vi "TWM Client Cmd Exec ADC Selfcalibration.vi"(7 "end of packet key":string="TWM:command:EndOfPacket", 8 "error in":errorcluster, 10 "timeout [s] (300)":dbl=300.0, 11 "handle":i32) -> (0 "error out":errorcluster, 3 "handle out":i32)   [LabVIEW 2020, in "TWM Client.lvlib"]
doc: "Executes digitizer selfcalibration routine, waits for completion. It is blocking operation, so the client and TWM will hangup untill operation is done or fails! Cannot be called while measurement is in progress!"
uses:
  TWM Client.lvlib
  infolib.lvlib
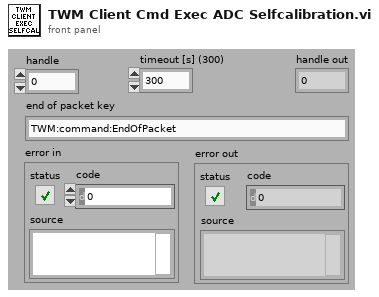
[diagram p1: front panel]
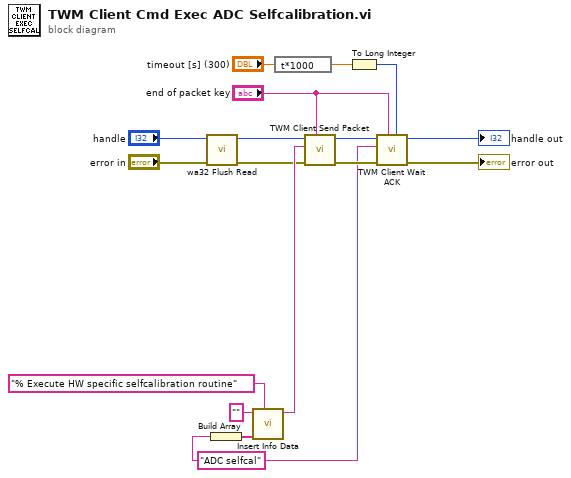
[diagram p0: block diagram]
diagram:
  w8 = "ADC selfcal" ("section name")
  n1 = call "wa32 Flush Read.vi"("error in"="error in", "handle"="handle") -> ("error out"=w3:errorcluster, "handle out"=w2:i32)  [unwired: 7 in, 1 out]
  n2 = Build Array(w8) -> (w16:string[])
  n3 = call "Insert Info Data.vi"("info data to insert"="% Execute HW specific selfcalibration routine", "sections"=w16, "info data"="") -> ("info data out"=w17:string)  [unwired: 7 in, 1 out]
  n4 = expression code="t*1000"("timeout [s] (300)") -> (w6:dbl)
  n5 = call "TWM Client Send Packet.vi"("end of packet key"="end of packet key", "error in"=w3, "command string"=w17, "handle"=w2) -> ("error out"=w14:errorcluster, "handle out"=w13:i32)  [unwired: 6 in]
  n6 = To Long Integer(number=w6) -> (32bit integer=w5:i32)
  n7 = call "TWM Client Wait ACK.vi"("timeout [ms] (3000)"=w5, "key string"="end of packet key", "error in"=w14, "command header"=w8, "handle"=w13) -> ("error out"=→"error out":errorcluster, "handle out"=→"handle out":i32)  [unwired: 5 in]
